vi "Initial_Value_Shift_Register.vi"() -> ()   [LabVIEW 2017]
panel:
  out "Indicator 2":dbl
  out "Indicator 1":dbl
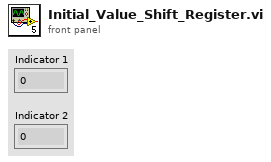
[diagram p1: front panel]
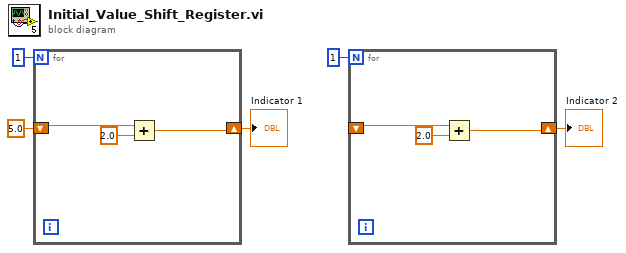
[diagram p0: block diagram]
diagram:
  n1 = for {
    N: 1 -> [_]
    shift-right: [w6] -> w3
    shift-left: 5.0 -> [w8]
    n2 = Add(x=w8, y=2.0) -> (x+y=w6:dbl)
  }
  "Indicator 1" <- w3
  n3 = for {
    N: 1 -> [_]
    shift-right: [w9] -> w2
    shift-left: _ -> [w11]
    n4 = Add(x=w11, y=2.0) -> (x+y=w9:dbl)
  }
  "Indicator 2" <- w2
